vi "FlatToRichcif_manager_PluginStatus.vi"(5 "OutputClusterType":T1, 11 "InputCluster":T15) -> (3 "OutputCluster":T1)   [LabVIEW 2021, in "CIF_Manager_server.lvlib"]
uses:
  CIF_Manager_server.lvlib
  cif_manager_PluginStatus_Flat.ctl
  cif_management_common_PluginStatusData_Flat.ctl
  cif_management_common_PluginStatusData_PluginState.ctl
  cif_management_common_TimingStatistics_Flat.ctl
  cif_common_TimingStats_Flat.ctl
  cif_management_common_FifoStatistics_Flat.ctl
  cif_management_common_Error_Flat.ctl
  cif_management_common_MonitorDoubles_Flat.ctl
  cif_management_common_MonitorU64_Flat.ctl
  cif_management_common_MonitorI64_Flat.ctl
  cif_management_common_Channels_Flat.ctl
  cif_management_common_Channel_Flat.ctl
  cif_management_common_ChannelDirection.ctl
  cif_management_common_ChannelPattern.ctl
  cif_manager_PluginStatus.ctl
  cif_management_common_PluginStatusData.ctl
  cif_management_common_TimingStatistics.ctl
  cif_common_TimingStats.ctl
  cif_management_common_FifoStatistics.ctl
  cif_management_common_Error.ctl
  cif_management_common_MonitorDoubles.ctl
  cif_management_common_MonitorU64.ctl
  cif_management_common_MonitorI64.ctl
  cif_management_common_Channels.ctl
  cif_management_common_Channel.ctl
  FlatToRichcif_management_common_TimingStatistics.vi
  FlatToRichcif_management_common_FifoStatistics.vi
  FlatToRichcif_management_common_Error.vi
  FlatToRichcif_management_common_MonitorDoubles.vi
  FlatToRichcif_management_common_MonitorU64.vi
  FlatToRichcif_management_common_MonitorI64.vi
  FlatToRichcif_management_common_Channel.vi
  FlatToRichcif_common_TimingStats.vi
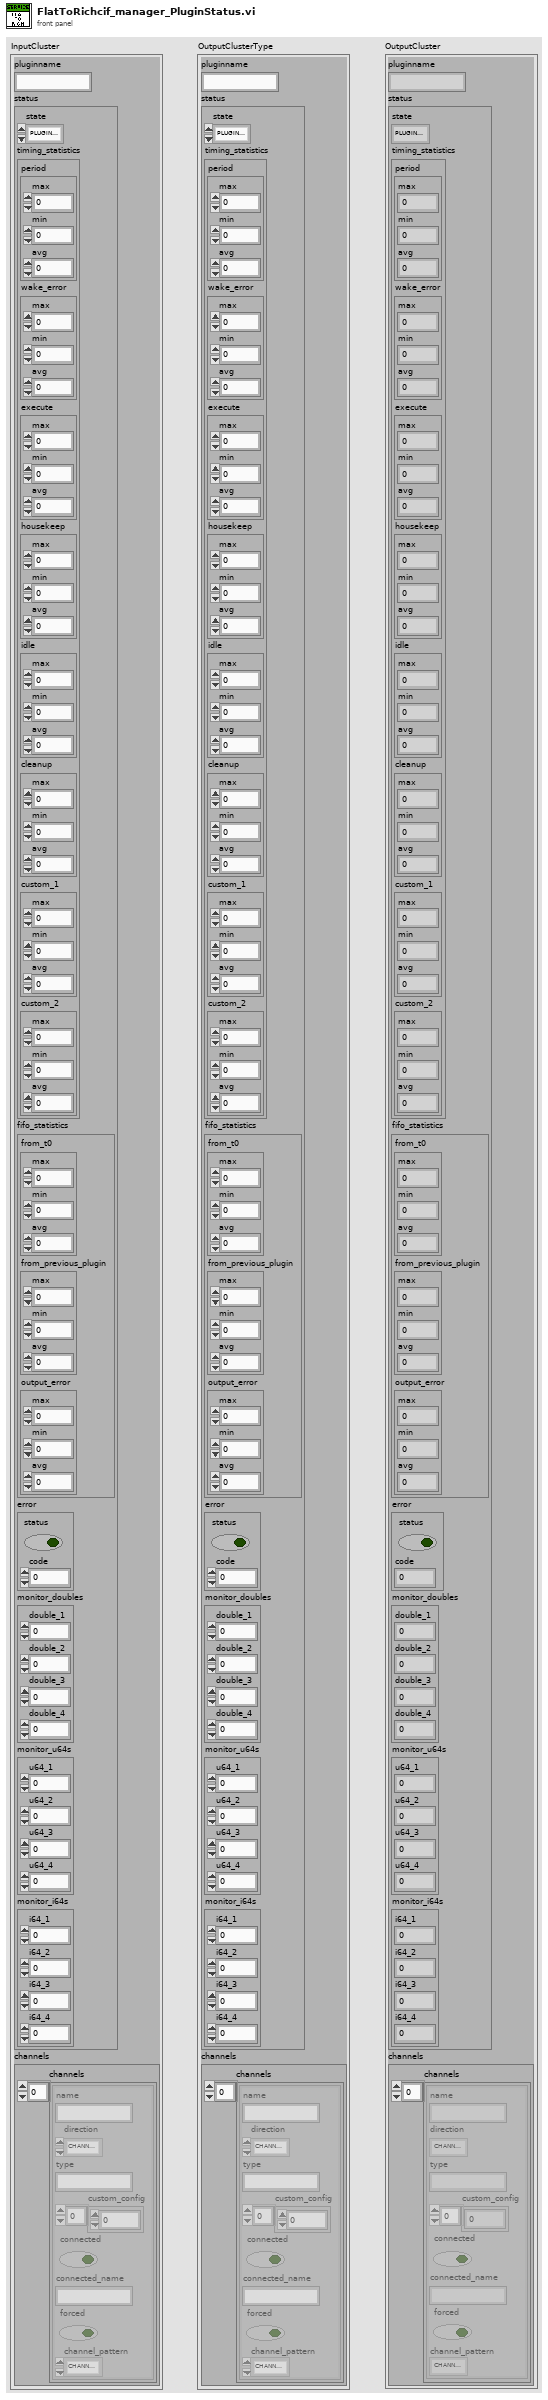
[diagram p1: front panel]
types:
  T1 = typedef "CIF_Manager_server.lvlib/cif_manager_PluginStatus.ctl" = cluster{"pluginname":string, "status":T2, "channels":T11}
  T2 = typedef "CIF_Manager_server.lvlib/cif_management_common_PluginStatusData.ctl" = cluster{"state":T3, "timing_statistics":T4, "fifo_statistics":T6, "error":T7, "monitor_doubles":T8, "monitor_u64s":T9, "monitor_i64s":T10}
  T3 = typedef "CIF_Manager_server.lvlib/cif_management_common_PluginStatusData_PluginState.ctl" = enum32{"PLUGINSTATE_UNKNOWN", "PLUGINSTATE_CREATING", "PLUGINSTATE_LISTENING", "PLUGINSTATE_RUNNING", "PLUGINSTATE_CLEANINGUP", "PLUGINSTATE_DESTROYING", "PLUGINSTATE_PREPARED", "PLUGINSTATE_FTE_RUN"}
  T4 = typedef "CIF_Manager_server.lvlib/cif_management_common_TimingStatistics.ctl" = cluster{"period":T5, "wake_error":T5, "execute":T5, "housekeep":T5, "idle":T5, "cleanup":T5, "custom_1":T5, "custom_2":T5}
  T5 = typedef "CIF_Manager_server.lvlib/cif_common_TimingStats.ctl" = cluster{"max":i64, "min":i64, "avg":dbl}
  T6 = typedef "CIF_Manager_server.lvlib/cif_management_common_FifoStatistics.ctl" = cluster{"from_t0":T5, "from_previous_plugin":T5, "output_error":T5}
  T7 = typedef "CIF_Manager_server.lvlib/cif_management_common_Error.ctl" = cluster{"status":bool, "code":i32}
  T8 = typedef "CIF_Manager_server.lvlib/cif_management_common_MonitorDoubles.ctl" = cluster{"double_1":dbl, "double_2":dbl, "double_3":dbl, "double_4":dbl}
  T9 = typedef "CIF_Manager_server.lvlib/cif_management_common_MonitorU64.ctl" = cluster{"u64_1":u64, "u64_2":u64, "u64_3":u64, "u64_4":u64}
  T10 = typedef "CIF_Manager_server.lvlib/cif_management_common_MonitorI64.ctl" = cluster{"i64_1":i64, "i64_2":i64, "i64_3":i64, "i64_4":i64}
  T11 = typedef "CIF_Manager_server.lvlib/cif_management_common_Channels.ctl" = cluster{"channels":T12[]}
  T12 = typedef "CIF_Manager_server.lvlib/cif_management_common_Channel.ctl" = cluster{"name":string, "direction":T13, "type":string, "custom_config":u8[], "connected":bool, "connected_name":string, "forced":bool, "channel_pattern":T14}
  T13 = typedef "CIF_Manager_server.lvlib/cif_management_common_ChannelDirection.ctl" = enum32{"CHANNELDIRECTION_UNKNOWN", "CHANNELDIRECTION_PUBLISHER", "CHANNELDIRECTION_SUBSCRIBER"}
  T14 = typedef "CIF_Manager_server.lvlib/cif_management_common_ChannelPattern.ctl" = enum32{"CHANNELPATTERN_UNKNOWN", "CHANNELPATTERN_TAG", "CHANNELPATTERN_FIFO", "CHANNELPATTERN_MULTIFIFO", "CHANNELPATTERN_BACKPRESSUREFIFO"}
  T15 = typedef "CIF_Manager_server.lvlib/cif_manager_PluginStatus_Flat.ctl" = cluster{"pluginname":string, "status":T16, "channels":T24}
  T16 = typedef "CIF_Manager_server.lvlib/cif_management_common_PluginStatusData_Flat.ctl" = cluster{"state":T3, "timing_statistics":T17, "fifo_statistics":T19, "error":T20, "monitor_doubles":T21, "monitor_u64s":T22, "monitor_i64s":T23}
  T17 = typedef "CIF_Manager_server.lvlib/cif_management_common_TimingStatistics_Flat.ctl" = cluster{"period":T18, "wake_error":T18, "execute":T18, "housekeep":T18, "idle":T18, "cleanup":T18, "custom_1":T18, "custom_2":T18}
  T18 = typedef "CIF_Manager_server.lvlib/cif_common_TimingStats_Flat.ctl" = cluster{"max":i64, "min":i64, "avg":dbl}
  T19 = typedef "CIF_Manager_server.lvlib/cif_management_common_FifoStatistics_Flat.ctl" = cluster{"from_t0":T18, "from_previous_plugin":T18, "output_error":T18}
  T20 = typedef "CIF_Manager_server.lvlib/cif_management_common_Error_Flat.ctl" = cluster{"status":bool, "code":i32}
  T21 = typedef "CIF_Manager_server.lvlib/cif_management_common_MonitorDoubles_Flat.ctl" = cluster{"double_1":dbl, "double_2":dbl, "double_3":dbl, "double_4":dbl}
  T22 = typedef "CIF_Manager_server.lvlib/cif_management_common_MonitorU64_Flat.ctl" = cluster{"u64_1":u64, "u64_2":u64, "u64_3":u64, "u64_4":u64}
  T23 = typedef "CIF_Manager_server.lvlib/cif_management_common_MonitorI64_Flat.ctl" = cluster{"i64_1":i64, "i64_2":i64, "i64_3":i64, "i64_4":i64}
  T24 = typedef "CIF_Manager_server.lvlib/cif_management_common_Channels_Flat.ctl" = cluster{"channels":T25[]}
  T25 = typedef "CIF_Manager_server.lvlib/cif_management_common_Channel_Flat.ctl" = cluster{"name":string, "direction":T13, "type":string, "custom_config":u8[], "connected":bool, "connected_name":string, "forced":bool, "channel_pattern":T14}
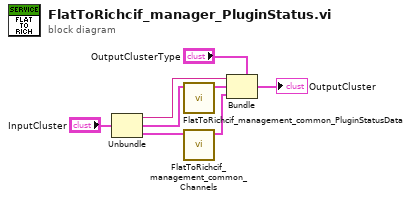
[diagram p0: block diagram]
diagram:
  n1 = Unbundle "Unbundle"("InputCluster") -> ("pluginname"=w5:string, "status"=w4:T16, "channels"=w2:T24)
  n2 = call "FlatToRichcif_management_common_PluginStatusData.vi"("InputCluster"=w4) -> ("OutputCluster"=w3:T2)  [unwired: 10 in]
  n3 = call "FlatToRichcif_management_common_Channels.vi"("InputCluster"=w2) -> ("OutputCluster"=w1:T11)  [unwired: 10 in]
  n4 = Bundle "Bundle"(cluster="OutputClusterType", "pluginname"=w5, "status"=w3, "channels"=w1) -> (→"OutputCluster":T1)
